vi "PDU Status.vi"(8 "error in":errorcluster) -> (0 "error out":errorcluster, 3 "OK":bool, 4 "PPS Status":T1, 5 "IP Status":string)   [LabVIEW 2023, in "HardwareAbstractionLayer_LVOOP.lvlib" / "Wait Monitor.lvclass"]
uses:
  Wait Monitor.lvclass
  Teststand Steptypes/GlobalVariable/GlobalVariableData.vi
  Wait Monitor.lvclass/Wait Monitor.ctl
  Database/Database.lvclass
  Teststand/Teststand.lvclass
  Teststand Steptypes/LTT_TeststandSteptypes.lvlib
  <userlib>/_OpenG.lib/error/error.llb/openg_error.lvlib
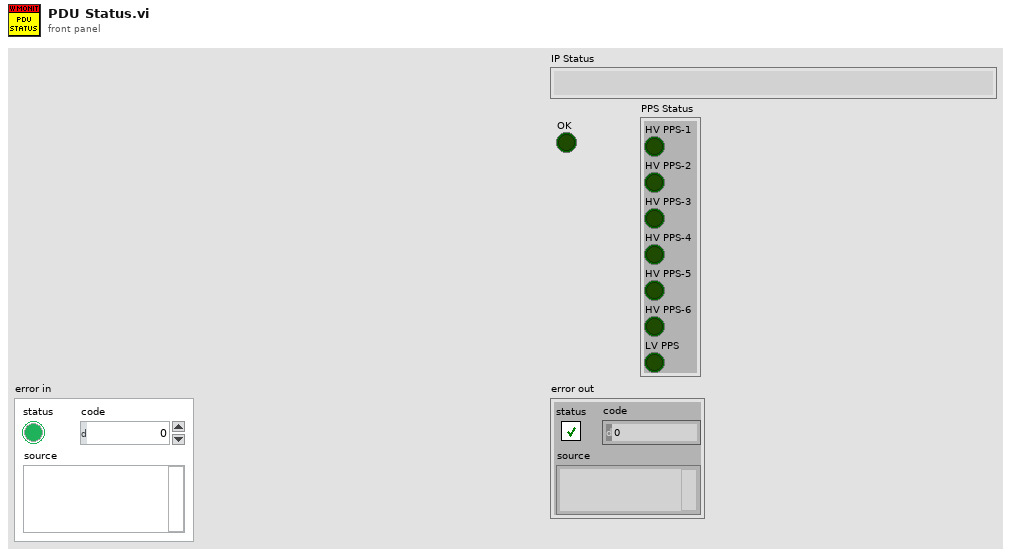
[diagram p1: front panel]
types:
  T1 = cluster{"HV PPS-1":bool, "HV PPS-2":bool, "HV PPS-3":bool, "HV PPS-4":bool, "HV PPS-5":bool, "HV PPS-6":bool, "LV PPS":bool}
  T2 = typedef "HardwareAbstractionLayer_LVOOP.lvlib/Teststand.lvclass/Teststand Status Control.ctl" = cluster{"Terminating or Aborting":bool, "Stop":bool, "Socket Count":i16, "Selected Sockets":i16[]}
  T3 = cluster{"[0]":bool, "[1]":bool, "[2]":bool, "[3]":bool, "[4]":bool, "[5]":bool, "[6]":bool}
  T4 = typedef "LTT_TeststandSteptypes.lvlib/PowerData.ctl" = cluster{"Chamber IP Ping":bool, "RAW_Power_Status":bool, "PDU1_Status_Instrument_Rack":bool, "PDU2_Status_PowerSupply_Rack_1":bool, "PDU3_Status_PowerSupply_Rack_2":bool}
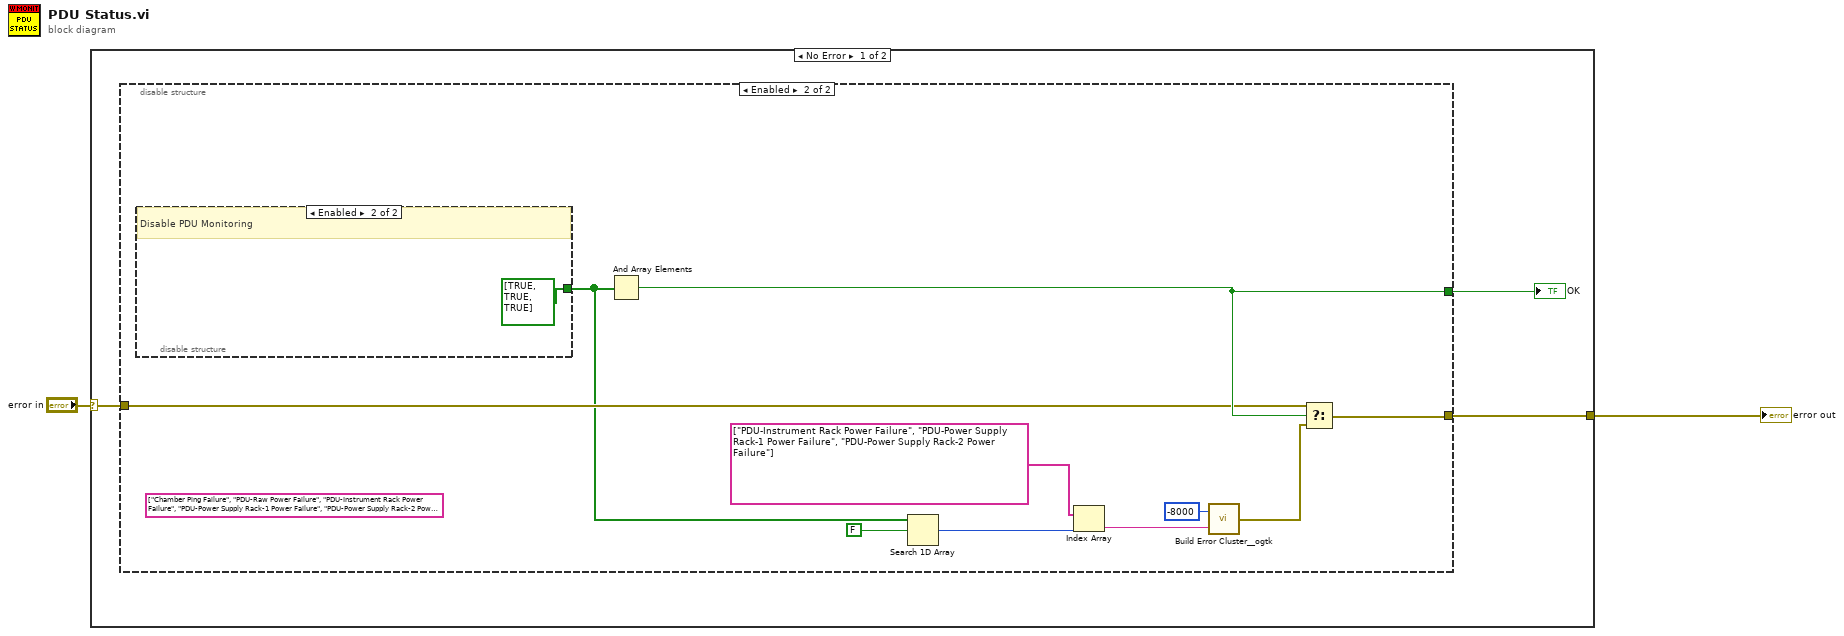
[diagram p0: block diagram]
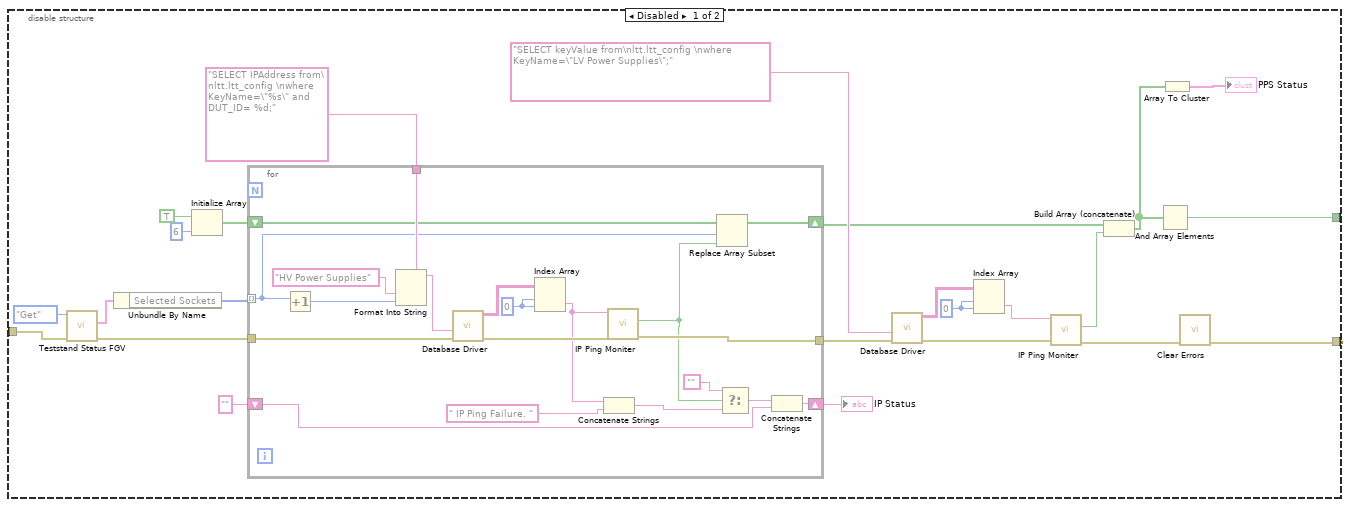
[diagram p2: hidden frame]
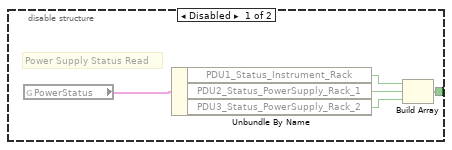
[diagram p3: hidden frame]
diagram:
  n1 = case shown="No Error" "error in" {
    selector: "error in" -> [w5 w66]
    tunnel: [w4 w66] -> w2
    frame No Error {
      n2 = disable-structure shown="Enabled" {
        disable-tunnel: w5 -> [w27 w57]
        disable-tunnel: [w18 w59] -> w4
        disable-tunnel: [w6 w58] -> w3
        frame Disabled {
          w22 = 0 ("index (row)")
          n3 = call "Teststand Status FGV.vi"("error in"=w27, "Option"=enum16{"Set", "Get"}."Get") -> ("error out"=w25:errorcluster, "Teststand Status Out"=w28:T2)  [unwired: 8 in]
          n4 = Unbundle By Name(w28) -> ("Selected Sockets"=w8:i16[])
          n5 = Initialize Array(TRUE, 6 ("dimension size")) -> (w12:bool[])
          n6 = for {
            tunnel: "SELECT IPAddress from\nltt.ltt_config \nwhere KeyName=\"%s\" and DUT_ID= %d;" -> [w48]
            tunnel: w25 -> [w47]
            tunnel: [w43] -> w20
            shift-right: [w40] -> w16
            shift-left: "" -> [w39]
            shift-right: [w31] -> w11
            shift-left: w12 -> [w33]
            tunnel: w8 -> [w30] mode=indexing
            w45 = 0 ("index (row)")
            n7 = Increment(x=w30) -> (x+1=w38:i16)
            n8 = Format Into String(format string=w48, "HV Power Supplies", w38) -> (resulting string=w36:string)  [unwired: 2 in, 1 out]
            n9 = call "Database Driver.vi"("error in"=w47, "SQL query"=w36) -> ("error out"=w44:errorcluster, "data"=w46:string[][])  [unwired: 6 in, 2 out]
            n10 = Index Array(array=w46, index (row)=w45, index (col)=w45) -> (element=w34:string)
            n11 = Concatenate Strings(w34, " IP Ping Failure. ") -> (w37:string)
            n12 = call "IP Ping Moniter.vi"("error in (no error)"=w44, "IP/Address"=w34) -> ("error out"=w43:errorcluster, "Sucessful?"=w32:bool)  [unwired: 7 in, 1 out]
            n13 = Replace Array Subset(array=w33, new element=w32, index=w30) -> (w31:bool[])
            n14 = Select(t="", s=w32, f=w37) -> (s? t:f=w41:string)
            n15 = Concatenate Strings(w41, w39) -> (w40:string)
          }
          "IP Status" <- w16
          n16 = call "Database Driver.vi"("error in"=w20, "SQL query"="SELECT keyValue from\nltt.ltt_config \nwhere KeyName=\"LV Power Supplies\";") -> ("error out"=w23:errorcluster, "data"=w21:string[][])  [unwired: 6 in, 2 out]
          n17 = Index Array(array=w21, index (row)=w22, index (col)=w22) -> (element=w24:string)
          n18 = call "IP Ping Moniter.vi"("error in (no error)"=w23, "IP/Address"=w24) -> ("error out"=w7:errorcluster, "Sucessful?"=w15:bool)  [unwired: 7 in, 1 out]
          n19 = Build Array (concatenate)(w11, w15) -> (w10:bool[])
          n20 = And Array Elements(Boolean array=w10) -> (logical AND=w6:bool)
          n21 = Array To Cluster(array=w10) -> (cluster=→"PPS Status":T3)
          n22 = call <vilib>:"Clear Errors.vi"("error in (no error)"=w7) -> ("error out"=w18:errorcluster)  [unwired: 5 in, 1 out]
        }
        frame Enabled {
          (unwired) string[] ["Chamber Ping Failure", "PDU-Raw Power Failure", "PDU-Instrument Rack Power Failure", "PDU-Power Supply Rack-1 Power Failure", "PDU-Power Supply Rack-2 Power Failure"]
          n23 = disable-structure shown="Enabled" {
            disable-tunnel: [w60 bool[] [TRUE, TRUE, TRUE]] -> w50
            frame Disabled {
              # "Power Supply Status Read"
              n24 = global read "GlobalVariableData.vi" "PowerStatus"() -> (w64:T4)
              n25 = Unbundle By Name(w64) -> ("PDU1_Status_Instrument_Rack"=w63:bool, "PDU2_Status_PowerSupply_Rack_1"=w62:bool, "PDU3_Status_PowerSupply_Rack_2"=w61:bool)
              n26 = Build Array(w63, w62, w61) -> (w60:bool[])
            }
            frame Enabled {
              # "Disable PDU Monitoring"
            }
          }
          n27 = And Array Elements(Boolean array=w50) -> (logical AND=w58:bool)
          n28 = Search 1D Array(1D array=w50, element=FALSE) -> (index of element=w55:i32)  [unwired: 1 in]
          n29 = Index Array(array=string[] ["PDU-Instrument Rack Power Failure", "PDU-Power Supply Rack-1 Power Failure", "PDU-Power Supply Rack-2 Power Failure"], index=w55) -> (element=w54:string)
          n30 = call <userlib>:"Build Error Cluster__ogtk.vi"("String to Prepend to source (\"\")"=w54, "code"=-8000) -> ("error out"=w53:errorcluster)
          n31 = Select(t=w57, s=w58, f=w53) -> (s? t:f=w59:errorcluster)
        }
      }
      "OK" <- w3
    }
    frame Error {
    }
  }
  "error out" <- w2
